vi "Confiugre Math Function FFT.vi"(7 "Window Function (0: Rectangular)":i32(ring) items=["Rectangular", "Hanning", "Flat Top", "Blackman-Harris"], 8 "error in (no error)":errorcluster, 9 "Frequency Span (100000.0 Hz)":dbl=100000.0, 10 "Center Frequency (50000.0 Hz)":dbl=50000.0, 11 "VISA resource name":refnum<visa-resource-name>) -> (0 "error out":errorcluster, 3 "VISA resource name out":refnum<visa-resource-name>)   [LabVIEW 2015, in "Agilent 2000 3000 X-Series.lvlib"]
doc: "Configures the math function FFT.\n\n<B>Note(s):</B>\nThis VI has been obsoleted from the driver and is included for compatibility with existing applications. New applications should use the <B>Configure Math Function (FFT) VI</B>."
uses:
  <instrlib>/Agilent 2000 3000 X-Series/Agilent 2000 3000 X-Series.lvlib
panel:
  # "Note:\nThis VI has been obsoleted from the driver and is included for compatibility with existing applications.  New applications should use the Configure Math Function (FFT) VI."
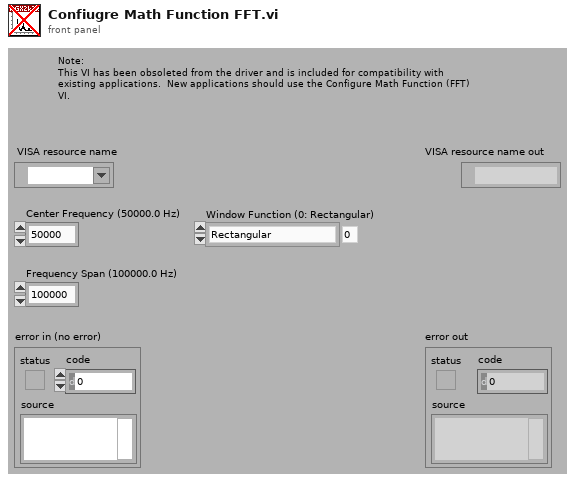
[diagram p1: front panel]
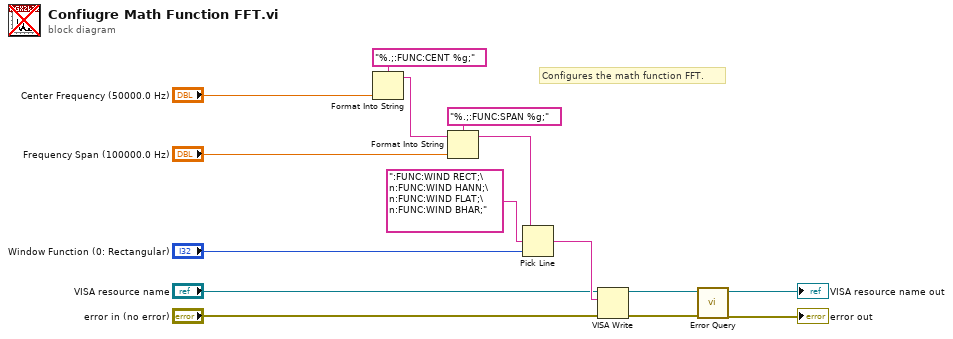
[diagram p0: block diagram]
diagram:
  # "Configures the math function FFT."
  n1 = Format Into String(format string="%.;:FUNC:CENT %g;", "Center Frequency (50000.0 Hz)") -> (resulting string=w13:string)  [unwired: 2 in, 1 out]
  n2 = Format Into String(format string="%.;:FUNC:SPAN %g;", initial string=w13, "Frequency Span (100000.0 Hz)") -> (resulting string=w8:string)  [unwired: 1 in, 1 out]
  n3 = Pick Line(string ("")=w8, multi-line string=":FUNC:WIND RECT;\n:FUNC:WIND HANN;\n:FUNC:WIND FLAT;\n:FUNC:WIND BHAR;", line index="Window Function (0: Rectangular)") -> (output string=w7:string)
  n4 = VISA Write(VISA resource name="VISA resource name", write buffer=w7, error in (no error)="error in (no error)") -> (VISA resource name out=w4:refnum<visa-resource-name>, error out=w3:errorcluster)  [unwired: 1 out]
  n5 = call <instrlib>:"Error Query.vi"("error in (no error)"=w3, "VISA resource name"=w4) -> ("error out"=→"error out":errorcluster, "VISA resource name out"=→"VISA resource name out":refnum<visa-resource-name>)  [unwired: 8 out]
